vi "ReadFromPannelAddressSpace.vi"(8 "error in (no error)":errorcluster, 11 "comms cluster in":T1) -> (0 "error out":errorcluster, 1 "input discrete":bool[](array[boolean]), 2 "input registers":u16[](array[numeric]), 3 "comms cluster out":T1, 4 "scratch input registers":u16[](array[numeric]))   [LabVIEW 2025]
doc: "Reads all input registers from MB server.\n\nINPUTS:\n 1. comms cluster of:\n a) station reg start address\n b)16-bit modulo of local user IP\n c) MB comms line \n 2. comms error line\n\nOUTPUTS:\n 1. repackaged comms cluster of:\n a) station reg start address\n b)16-bit modulo of local user IP\n c) MB comms line \n 2. comms error line\n 3. Input registers -- MB server registers\n associated with phys. pannel inputs\n (from pannel)\n 4. Input discretes -- MB server discrete\n storage read -- MB memory associated\n with physical pannel digital inputs.\n 5. Scratch input registers -- MB server\n registers associated with interapplication\n comms. -- e.g.: transaction of information\n between MATLAB and this VI."
uses:
  <vilib>/Modbus/master/Modbus Master.lvclass
panel:
  # "Read all pannel registers and contacts\n\nReads all input registers from MB server.\n\nINPUTS:\n  1. comms cluster of:\n      a) station reg start address\n      b)16-bit modulo of local user IP\n      c) MB comms line \n   2. comms error line\n\nOUTPUTS:\n   1. repackaged comms cluster of:\n      a) station reg start address\n      b)16-bit modulo of local user IP\n      c) MB comms line \n   2. comms error line\n   3. Input registers -- MB server registers\n       associated with phys. pannel inputs\n       (from pannel)\n   4. Input discretes -- MB server discrete\n       storage read -- MB memory associated\n       with physical pannel digital inputs.\n   5. Scratch input registers -- MB server\n       registers associated with interapplication\n       comms. -- e.g.: transaction of information\n       between MATLAB and this VI."
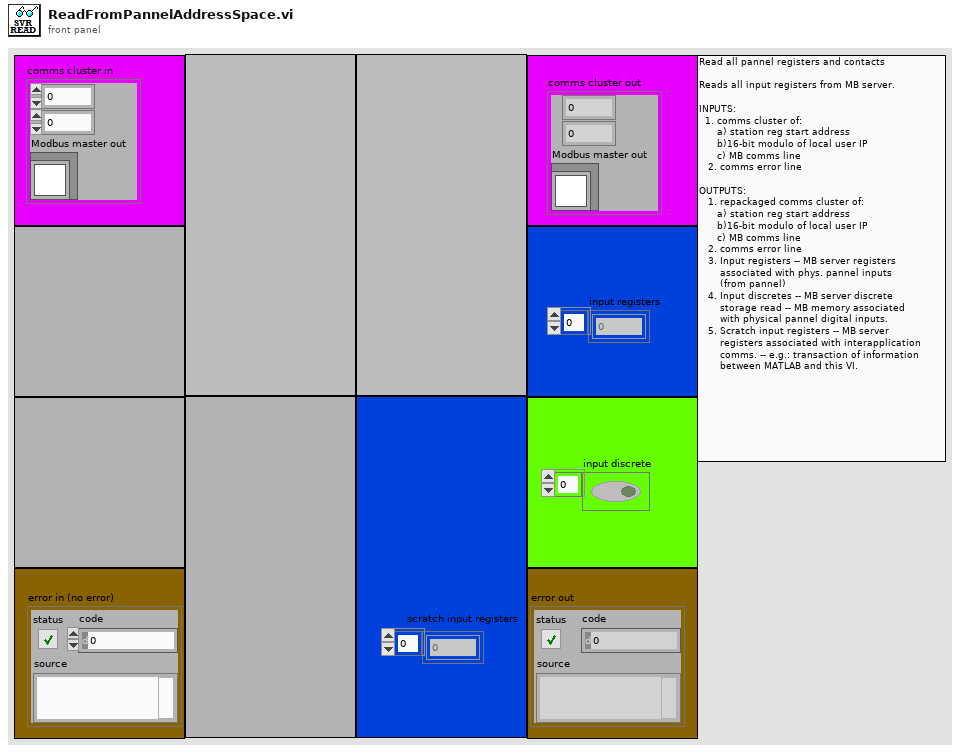
[diagram p1: front panel]
types:
  T1 = cluster{u16, u32, "Modbus master out":refnum<class "Modbus Master.lvclass">}
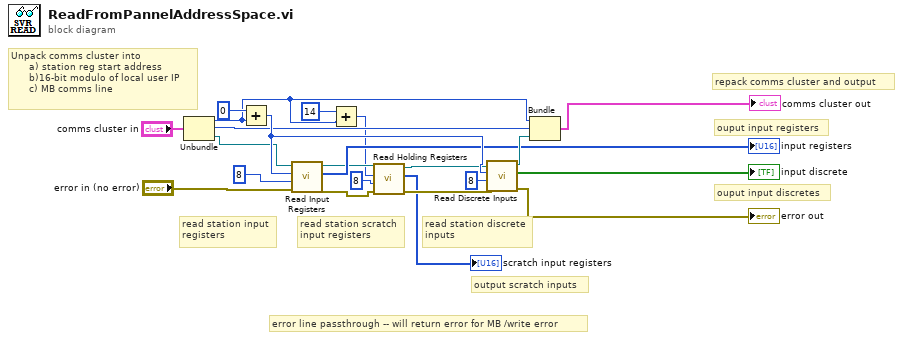
[diagram p0: block diagram]
diagram:
  # "ouput input discretes"
  # "ouput input registers"
  # "repack comms cluster and output"
  # "Unpack comms cluster into\n      a) station reg start address\n      b)16-bit modulo of local user IP\n      c) MB comms line"
  # "error line passthrough -- will return error for MB /write error"
  # "output scratch inputs"
  # "read station discrete\ninputs"
  # "read station scratch\ninput registers"
  # "read station input\nregisters"
  n1 = Unbundle("comms cluster in") -> (w8:u16, w10:u32, "Modbus master out"=w15:refnum<class "Modbus Master.lvclass">)
  n2 = Add(x=u16 0, y=w8) -> (x+y=w18:u16)
  n3 = call-dynamic "Read Input Registers.vi"("error in (no error)"="error in (no error)", "number of input registers"=u16 8 ("number of holding registers"), "starting address"=w18, "Modbus master in"=w15) -> ("error out"=w4:errorcluster, "register values"=→"input registers":u16[], "Modbus master out"=w3:refnum<class "Modbus Master.lvclass">)  [unwired: 5 in]
  n4 = Add(x=u16 14, y=w8) -> (x+y=w2:u16)
  n5 = call-dynamic "Read Holding Registers.vi"("error in (no error)"=w4, "number of holding registers"=u16 8 ("number of discrete inputs"), "starting address"=w2, "Modbus master in"=w3) -> ("error out"=w7:errorcluster, "register values"=→"scratch input registers":u16[], "Modbus master out"=w6:refnum<class "Modbus Master.lvclass">)  [unwired: 5 in]
  n6 = call-dynamic "Read Discrete Inputs.vi"("error in (no error)"=w7, "number of discrete inputs"=u16 8, "starting address"=w18, "Modbus master in"=w6) -> ("error out"=→"error out":errorcluster, "discrete input values"=→"input discrete":bool[], "Modbus master out"=w20:refnum<class "Modbus Master.lvclass">)  [unwired: 5 in]
  n7 = Bundle(w8, w10, "Modbus master out"=w20) -> (→"comms cluster out":T1)  [unwired: 1 in]
